vi "PXI-Set DAQ In Progress Global.vi"(0 "In progress?":bool, 11 "error in (no error)":errorcluster) -> (4 "In progress (out)":bool, 15 "error out":errorcluster)   [LabVIEW 2020]
uses:
  PXI Globals.vi
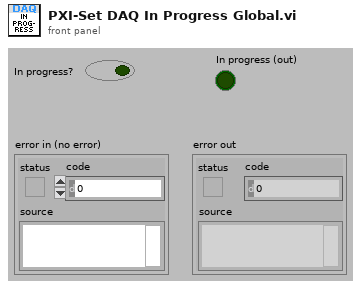
[diagram p1: front panel]
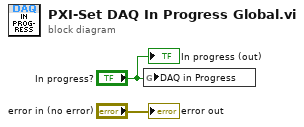
[diagram p0: block diagram]
diagram:
  n1 = global write "PXI Globals.vi" "DAQ in Progress"("In progress?") -> ()
  "error out" <- "error in (no error)"
  "In progress (out)" <- "In progress?"
